vi "setTargetState (byObject).vi"(8 "error in (no error)":errorcluster, 10 "Target State":refnum<class "state.lvclass">, 11 "State":refnum<class "state.lvclass">) -> (0 "error out":errorcluster, 2 "Target State dup":refnum<class "state.lvclass">, 3 "State out":refnum<class "state.lvclass">)   [LabVIEW 2020, in "eos.lvlib" / "state.lvclass"]
uses:
  state.lvclass
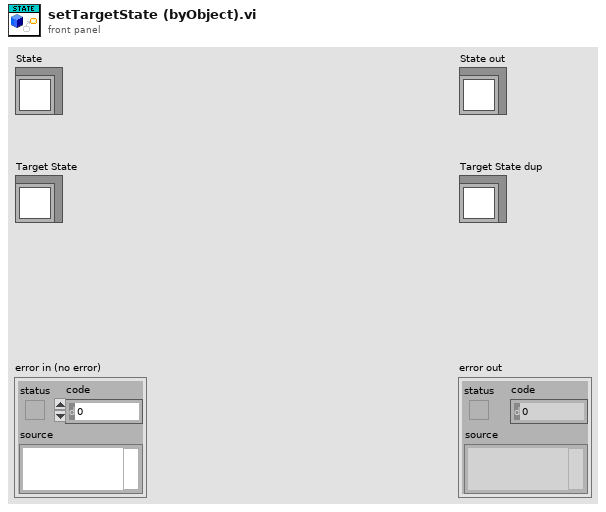
[diagram p1: front panel]
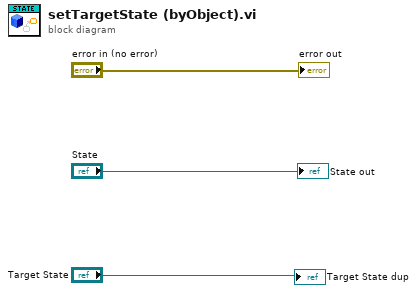
[diagram p0: block diagram]
diagram:
  "error out" <- "error in (no error)"
  "State out" <- "State"
  "Target State dup" <- "Target State"
